vi "refereeToGUIReferee.vi"(6 "Command":string, 8 "error in (no error)":errorcluster, 10 "SSL Game Status":T2, 11 "Vision in":refnum<class "Vision.lvclass">) -> (0 "error out":errorcluster, 1 "SSL Referee Game Status":T1 {"Time" format="%<%.3X %x>T"; "Blue Timeout Remaining" format="%<%M:%S>t"; "Yellow Timeout Remaining" format="%<%M:%S>t"; "Time Left" format="%<%M:%S>t"}, 2 "GUI Game Status":T1 {"Time" format="%<%.3X %x>T"; "Blue Timeout Remaining" format="%<%M:%S>t"; "Yellow Timeout Remaining" format="%<%M:%S>t"; "Time Left" format="%<%M:%S>t"}, 3 "Vision out":refnum<class "Vision.lvclass">)   [LabVIEW 2023, in "Vision.lvclass"]
uses:
  Vision.lvclass
  Old vision/Decode SSL and Refree Wrapper Package Folder/SSL Referee Game Status.ctl
  Old vision/Controls/SSL Referee.ctl
  Old vision/Decode SSL and Refree Wrapper Package Folder/SSL Referee Team Info.ctl
panel:
  # "Score"
  # "Red Cards"
  # "Yellow Cards"
  # "Timeouts Left"
  # "Timeout Remaining"
  # "Goalie ID"
  # "Score"
  # "Red Cards"
  # "Yellow Cards"
  # "Timeouts Left"
  # "Timeout Remaining"
  # "Goalie ID"
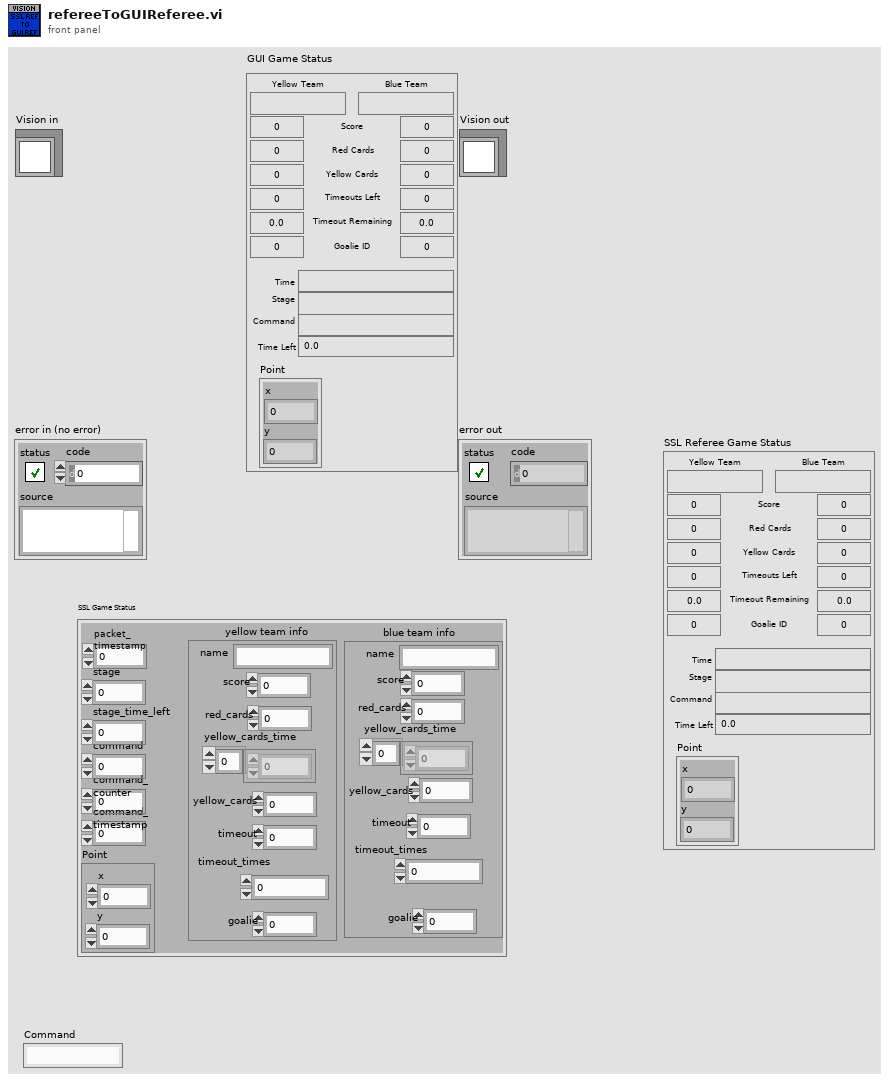
[diagram p1: front panel]
types:
  T1 = typedef "SSL Referee Game Status.ctl" = cluster{"Stage":string, "Command":string, "Time Left":dbl, "Yellow Team":string, "Blue Team":string, "Yellow Score":u32, "Blue Score":u32, "Yellow Red Cards":u32, "Blue Red Cards":u32, "Yellow Yellow Cards":u32, "Blue Yellow Cards":u32, "Yellow Timeouts Left":u32, "Blue Timeouts Left":u32, "Yellow Timeout Remaining":dbl, "Blue Timeout Remaining":dbl, "Yellow Goalie Id":u32, "Blue Goalie Id":u32, "Time":timestamp, "Point":cluster{"x":sgl, "y":sgl}}
  T2 = typedef "SSL Referee.ctl" = cluster{"packet_\ntimestamp":u64, "stage":u64, "stage_time_left":i32, "command ":u64, "command_\ncounter ":u32, "command_\ntimestamp":u64, "yellow team info":T3, "blue team info":T3, "Point":cluster{"x":sgl, "y":sgl}}
  T3 = typedef "SSL Referee Team Info.ctl" = cluster{"name":string, "score":u32, "red_cards":u32, "yellow_cards_time":u32[], "yellow_cards":u32, "timeout":u32, "timeout_times":u32, "goalie":u32}
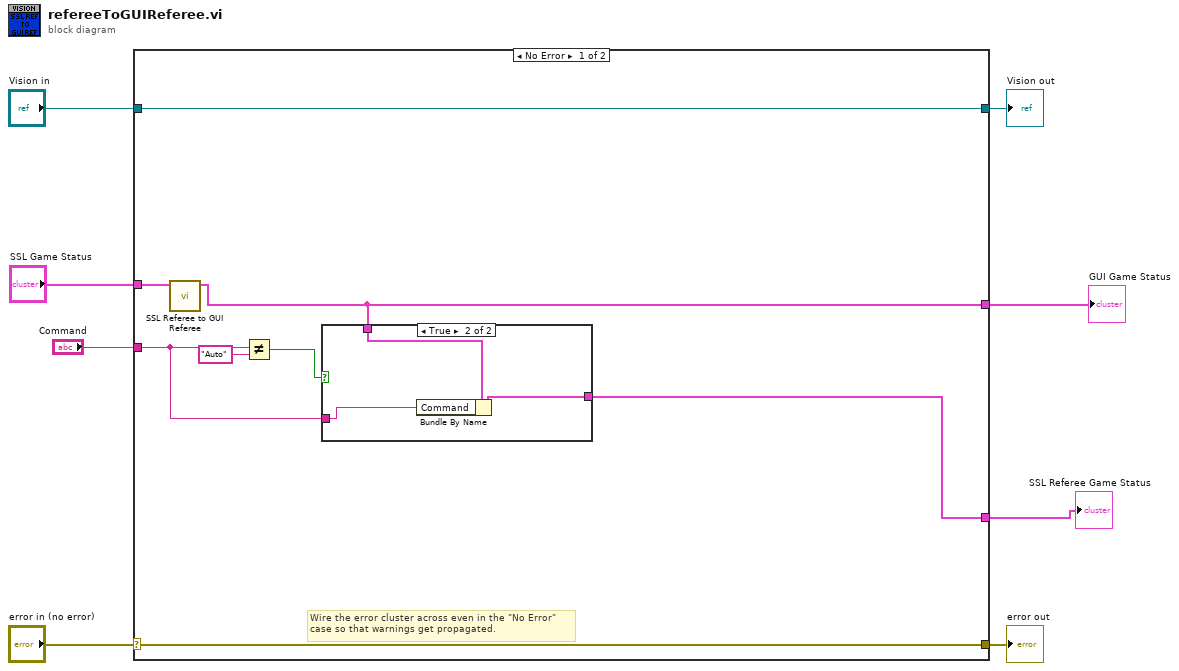
[diagram p0: block diagram]
diagram:
  n1 = case shown="No Error" "error in (no error)" {
    selector: "error in (no error)" -> [w15 w22]
    tunnel: [w15 w22] -> w7
    tunnel: [w16 w21] -> w5
    tunnel: "Vision in" -> [w16 w21]
    tunnel: "SSL Game Status" -> [w9 _]
    tunnel: [w12 _] -> w3
    tunnel: "Command" -> [w11 _]
    tunnel: [w10 _] -> w1
    frame No Error {
      # "Wire the error cluster across even in the \"No Error\"\ncase so that warnings get propagated."
      n2 = call "SSL Referee to GUI Referee.vi"("SSL Game Status"=w9) -> ("GUI Game Status"=w12:T1)  [unwired: 10 in]
      n3 = Not Equal?(x=w11, y="Auto") -> (x != y?=w13:bool)
      n4 = case shown="True" w13 {
        tunnel: [w17 w19] -> w10
        tunnel: w12 -> [w17 w20]
        tunnel: w11 -> [_ w18]
        frame False {
        }
        frame True {
          n5 = Bundle By Name(cluster=w20, "Command"=w18) -> (w19:T1)
        }
      }
    }
    frame Error {
    }
  }
  "error out" <- w7
  "Vision out" <- w5
  "GUI Game Status" <- w3
  "SSL Referee Game Status" <- w1
